vi "WHH Formula.vi"(4 "data":variant, 5 "x":dbl) -> (2 "WHH(x)":dbl format="%.19f")   [LabVIEW 2021]
uses:
  WHH Formula Data.ctl
  <vilib>/gmath/NI_Gmath.lvlib
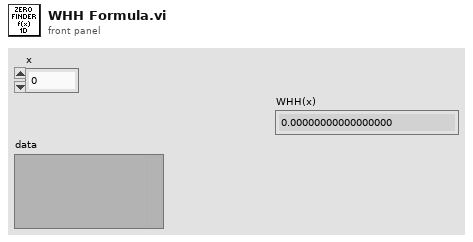
[diagram p1: front panel]
types:
  T1 = typedef "WHH Formula Data.ctl" = cluster{"t":dbl, "alpha_Maki":dbl, "lambda_SO":dbl}
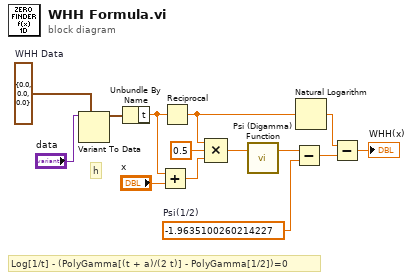
[diagram p0: block diagram]
diagram:
  w6 = -1.9635100260214227  # Psi(1/2)
  w13 = T1 {"t"=0.0, "alpha_Maki"=0.0, "lambda_SO"=0.0}  # WHH Data
  # "h"
  # "Log[1/t] - (PolyGamma[(t + a)/(2 t)] - PolyGamma[1/2])=0"
  n1 = Variant To Data(type=w13, Variant="data") -> (data=w8:T1)  [unwired: 1 in, 1 out]
  n2 = Unbundle By Name(w8) -> ("t"=w7:dbl)
  n3 = Add(x=w7, y="x") -> (x+y=w12:dbl)
  n4 = Reciprocal(x=w7) -> (1/x=w11:dbl)
  n5 = Compound Arithmetic op=MULTIPLY(w11, 0.5, w12) -> (w10:dbl)
  n6 = call <vilib>:"Psi (Digamma) Function.vi"("x"=w10) -> ("y(x)"=w5:dbl)  [unwired: 2 in]
  n7 = Subtract(x=w5, y=w6) -> (x-y=w3:dbl)
  n8 = Natural Logarithm(1:w11) -> (0:w4:dbl)
  n9 = Subtract(x=w4, y=w3) -> (x-y=→"WHH(x)":dbl)
